vi "Alerts.vi"(0 "IP":string="localhost", 1 "ID":u8, 2 "EnRefnum":refnum<vi>, 3 "StRefnum":refnum<vi>, 5 "Port":u16=6341, 11 "error in (no error)":errorcluster) -> (15 "error out":errorcluster)   [LabVIEW 2011]
uses:
  LVOOP/Ethernet/TCP Alerts/TCPAlerts.lvclass
  Variable/gSTOP.vi
  Queue/Alert.vi
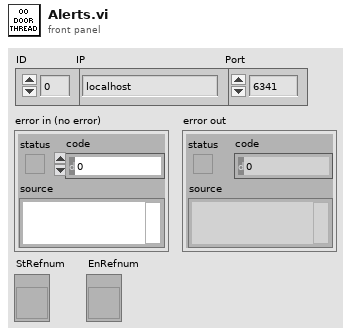
[diagram p1: front panel]
types:
  T1 = enum16{"Open", "R", "W", "R->W", "W->R", "Close"}
  T2 = enum16{"Obtain", "Enqueue", "Dequeue", "Release"}
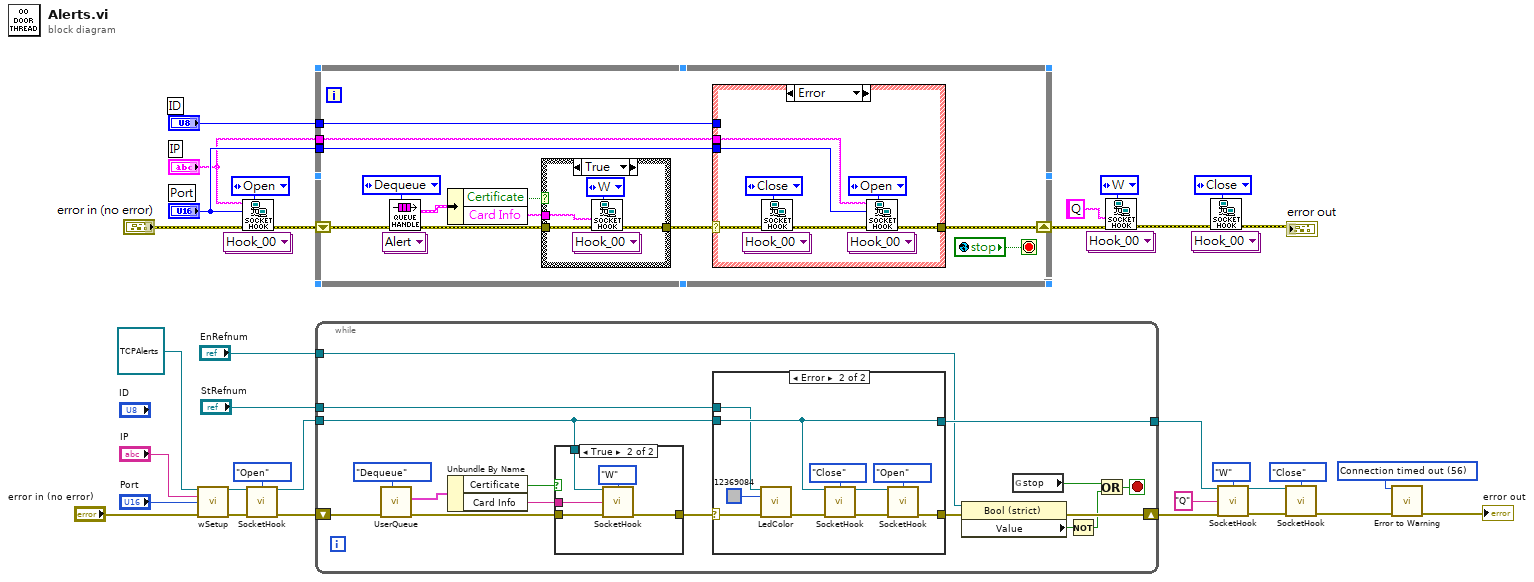
[diagram p0: block diagram]
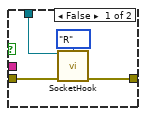
[diagram p2: hidden frame]
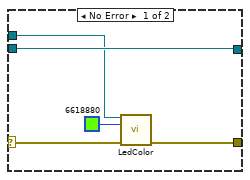
[diagram p3: hidden frame]
diagram:
  w3 = 56 items=["No Error", "Argument Error", "Memory Full", "Out of Zone", "End of File", "File Already Open", "Generic File IO Error", "File Not Found", "File Permission Error", "Disk Full", "Duplicate Path", "Too Many Files Open", "Not Enabled", "Resource File Not Found", "Cannot Add Resource", "Resource Not Found", "Image Not Found", "Image Memory Error", "Pen Does Not Exist", "Config Bad Type", "Config Token Not Found", "Config Parse Error", "Config Memory Error", "Bad External Code Format", "Bad External Code Offset", "External Code Not Present", "Null Window", "Destroy Window Mixup", "Null Menu", "Print Aborted", "Bad Print Record", "Print Driver Error", "Windows Error During Print", "Memory Error During Print", "Print Dialog Error", "Generic Print Error", "Invalid Device Refnum", "Device Not Found", "Device Parameter Error", "Device Unit Error", "Can't Open Device", "Device Call Aborted", "Generic Error", "Cancelled By User", "Object ID Too Low", "Object ID Too High", "Object Not In Heap", "Unknown Heap", "Bad DefProc ID", "DefProc Not In Table", "Message Out Of Range", "Null Method", "Unknown Message", "Manager Call Not Supported", "Bad address", "Connection In progress", "Connection timed out", "Connection is already in progress", "Network attribute not supported", "Network error", "Address in use", "System out of memory", "Connection aborted", "Connection refused", "Connection is not connected", "Connection is already connected", "Connection closed", "Initialize error (interapplication manager)", "Bad occurrence", "Wait on unbound occurrence handler", "Occurrence queue overflow", "Bad path", "Semaphore not signaled", "Unrecognized type (interapplication manager)"] ("1st Error to Convert")
  n1 = call-dynamic "wSetup.vi"("Socket_000 in"=refnum<class "TCPAlerts.lvclass"> refnum ("Socket_000.lvclass"), "IP Address"="IP", "Port"="Port", "error in (no error)"="error in (no error)") -> ("Socket_000 out"=w11:refnum<class "TCPAlerts.lvclass">, "error out"=w10:errorcluster)  [unwired: 10 in]
  n2 = call-dynamic "SocketHook.vi"("Socket_000 in"=w11, "Mode"=T1."Open", "error in (no error)"=w10) -> ("Socket_000 out"=w8:refnum<class "TCPAlerts.lvclass">, "error out"=w9:errorcluster)  [unwired: 10 in, 1 out]
  n3 = while {
    shift-right: [w25] -> w18
    shift-left: w9 -> [w35]
    tunnel: w8 -> [w33]
    tunnel: [w32] -> w7
    tunnel: "StRefnum" -> [w31]
    tunnel: "EnRefnum" -> [w28]
    stop <- w22 stop-if-true
    n4 = call-poly "UserQueue.vi"("Mode"=T2."Dequeue", "error in (no error)"=w35) -> ("error out"=w38:errorcluster, "Queue Out"=w29:cluster{"Certificate":bool, "Card Info":string})  [unwired: 8 in]
    n5 = Unbundle By Name(w29) -> ("Certificate"=w37:bool, "Card Info"=w36:string)
    n6 = case shown="True" w37 {
      tunnel: [w40 w46] -> w34
      tunnel: w38 -> [w41 w45]
      tunnel: w36 -> [_ w44]
      tunnel: w33 -> [w39 w43]
      frame False {
        n7 = call-dynamic "SocketHook.vi"("Socket_000 in"=w39, "Mode"=T1."R", "error in (no error)"=w41) -> ("error out"=w40:errorcluster)  [unwired: 10 in, 2 out]
      }
      frame True {
        n8 = call-dynamic "SocketHook.vi"("Socket_000 in"=w43, "Mode"=T1."W", "data in"=w44, "error in (no error)"=w45) -> ("error out"=w46:errorcluster)  [unwired: 9 in, 2 out]
      }
    }
    n9 = case shown="Error" w34 {
      selector: w34 -> [w50 w55]
      tunnel: [w49 w61] -> w27
      tunnel: w33 -> [w52 w57]
      tunnel: [w52 w57] -> w32
      tunnel: w31 -> [w48 w53]
      frame No Error {
        n10 = call "LedColor.vi"("Boolean in"=w48, "Color Box"=u32 6618880, "error in (no error)"=w50) -> ("error out"=w49:errorcluster)  [unwired: 12 in]
      }
      frame Error {
        n11 = call "LedColor.vi"("Boolean in"=w53, "Color Box"=u32 12369084, "error in (no error)"=w55) -> ("error out"=w54:errorcluster)  [unwired: 12 in]
        n12 = call-dynamic "SocketHook.vi"("Socket_000 in"=w57, "Mode"=T1."Close", "error in (no error)"=w54) -> ("Socket_000 out"=w58:refnum<class "TCPAlerts.lvclass">, "error out"=w62:errorcluster)  [unwired: 10 in, 1 out]
        n13 = call-dynamic "SocketHook.vi"("Socket_000 in"=w58, "Mode"=T1."Open", "error in (no error)"=w62) -> ("error out"=w61:errorcluster)  [unwired: 10 in, 2 out]
      }
    }
    n14 = property class="Bool (strict)"(reference=w28, error in=w27) -> (error out=w25:errorcluster, "Value"=w26:bool)  [unwired: 1 out]
    n15 = global read "gSTOP.vi" "stop"() -> (w24:bool)
    n16 = Not(x=w26) -> (.not. x?=w23:bool)
    n17 = Or(x=w24, y=w23) -> (x .or. y?=w22:bool)
  }
  n18 = call-dynamic "SocketHook.vi"("Socket_000 in"=w7, "Mode"=T1."W", "data in"="Q", "error in (no error)"=w18) -> ("Socket_000 out"=w6:refnum<class "TCPAlerts.lvclass">, "error out"=w17:errorcluster)  [unwired: 9 in, 1 out]
  n19 = call-dynamic "SocketHook.vi"("Socket_000 in"=w6, "Mode"=T1."Close", "error in (no error)"=w17) -> ("error out"=w2:errorcluster)  [unwired: 10 in, 2 out]
  n20 = call <vilib>:"Error to Warning.vi"("1st Error to Convert"=w3, "error in"=w2) -> ("warning out"=→"error out":errorcluster)  [unwired: 3 in, 10 out]
